vi "Reconnect and Disconnect.vi"() -> ()   [LabVIEW 2018]
uses:
  TwinCAT ADS Class/Controls/Connection Information.ctl
  TwinCAT ADS Class/Controls/Address.ctl
  TwinCAT ADS Class/Controls/Connection Protocol.ctl
  TwinCAT ADS Class/Controls/Router State.ctl
  TwinCAT ADS Class/Controls/Connection State.ctl
  TwinCAT ADS Class/TwinCAT ADS.lvclass
panel:
  in  "stop":bool
  in  "Disconnect":bool
  in  "Reconnect":bool
  out "Connection Information":T1
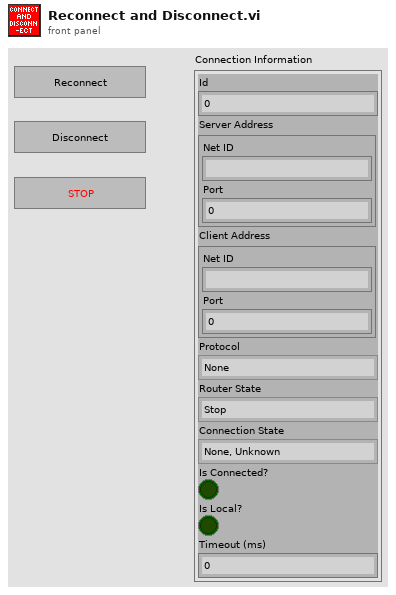
[diagram p1: front panel]
types:
  T1 = typedef "TwinCAT ADS.lvclass/Connection Information.ctl" = cluster{"Id":i32, "Server Address":T2, "Client Address":cluster{"Net ID":string, "Port":i32}, "Protocol":T3, "Router State":T4, "Connection State":T5, "Is Connected?":bool, "Is Local?":bool, "Timeout (ms)":i32}
  T2 = typedef "TwinCAT ADS.lvclass/Address.ctl" = cluster{"Net ID":string, "Port":i32}
  T3 = typedef "TwinCAT ADS.lvclass/Connection Protocol.ctl" = enum16{"None", "Router", "TCP/IP", "All"}
  T4 = typedef "TwinCAT ADS.lvclass/Router State.ctl" = enum16{"Stop", "Start", "Removed", "Unknown"}
  T5 = typedef "TwinCAT ADS.lvclass/Connection State.ctl" = enum16{"None, Unknown", "Disconnected", "Connected", "Lost"}
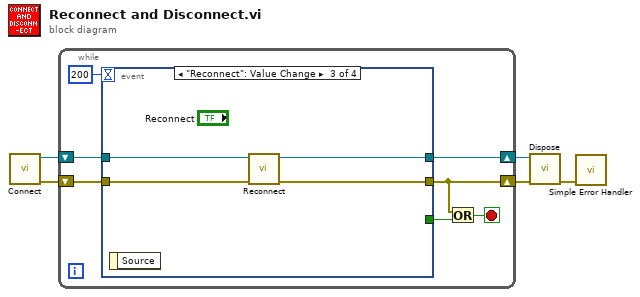
[diagram p0: block diagram]
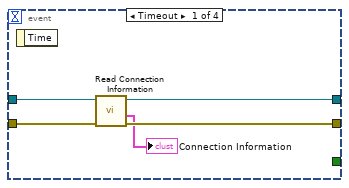
[diagram p2: hidden frame]
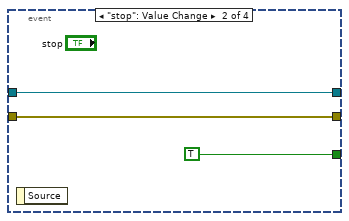
[diagram p3: hidden frame]
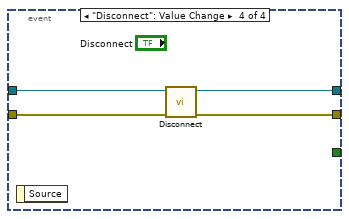
[diagram p4: hidden frame]
diagram:
  n1 = call "Connect.vi"() -> ("error out"=w5:errorcluster, "TwinCAT ADS out"=w4:refnum<class "TwinCAT ADS.lvclass">)  [unwired: 10 in]
  n2 = while {
    shift-right: [w10] -> w3
    shift-left: w4 -> [w12]
    shift-right: [w9] -> w2
    shift-left: w5 -> [w11]
    stop <- w6 stop-if-true
    n3 = event shown="[2] \"Reconnect\": Value Change" {
      selector: _ -> [_ _ _ _]
      dyn-events: _ -> [_ _ _ _]
      timeout: 200 -> [_ _ _ _]
      tunnel: w12 -> [w17 w20 w24 w27]
      tunnel: w11 -> [w16 w19 w23 w28]
      tunnel: [w14 w20 w21 w25] -> w10
      tunnel: [w15 w19 w22 w26] -> w9
      tunnel: [_ TRUE _ _] -> w7
      event Timeout {
        n4 = event-data() -> ()  [unwired: 1 in, 1 out]
        n5 = call "Read Connection Information.vi"("error in (no error)"=w16, "TwinCAT ADS in"=w17) -> ("error out"=w15:errorcluster, "Connection Information"=→"Connection Information":T1, "TwinCAT ADS out"=w14:refnum<class "TwinCAT ADS.lvclass">)  [unwired: 7 in]
      }
      event "stop": Value Change {
        n6 = event-data() -> ()  [unwired: 1 in, 1 out]
      }
      event "Reconnect": Value Change {
        n7 = event-data() -> ()  [unwired: 1 in, 1 out]
        n8 = call "Reconnect.vi"("error in (no error)"=w23, "TwinCAT ADS in"=w24) -> ("error out"=w22:errorcluster, "TwinCAT ADS out"=w21:refnum<class "TwinCAT ADS.lvclass">)  [unwired: 8 in]
      }
      event "Disconnect": Value Change {
        n9 = event-data() -> ()  [unwired: 1 in, 1 out]
        n10 = call "Disconnect.vi"("error in (no error)"=w28, "TwinCAT ADS in"=w27) -> ("error out"=w26:errorcluster, "TwinCAT ADS out"=w25:refnum<class "TwinCAT ADS.lvclass">)  [unwired: 7 in, 1 out]
      }
    }
    n11 = Or(x=w9, y=w7) -> (x .or. y?=w6:bool)
  }
  n12 = call "Dispose.vi"("error in (no error)"=w2, "TwinCAT ADS in"=w3) -> ("error out"=w1:errorcluster)  [unwired: 9 in]
  n13 = call <vilib>:"Simple Error Handler.vi"("error in (no error)"=w1) -> ()  [unwired: 4 in, 5 out]
